vi "rd_ser.vi"(3 "error in":errorcluster, 5 "VISA resource name in":refnum<visa-resource-name>) -> (0 "error out":errorcluster, 1 "read buffer":string, 2 "VISA resource name out":refnum<visa-resource-name>)   [LabVIEW 2010]
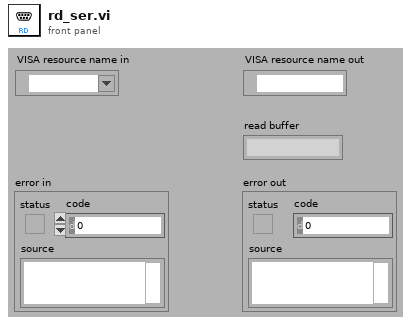
[diagram p1: front panel]
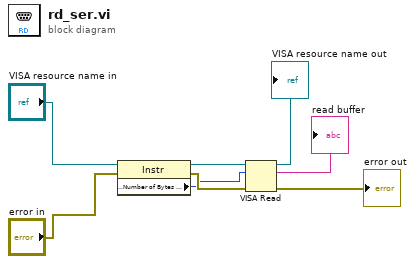
[diagram p0: block diagram]
diagram:
  n1 = property class="Instr"(reference="VISA resource name in", error in="error in") -> (reference out=w3:refnum<visa-resource-name>, error out=w2:errorcluster, "Serial Settings:Number of Bytes at Serial Port"=w1:u32)
  n2 = VISA Read(VISA resource name=w3, byte count=w1, error in (no error)=w2) -> (VISA resource name out=→"VISA resource name out":refnum<visa-resource-name>, read buffer=→"read buffer":string, error out=→"error out":errorcluster)  [unwired: 1 out]
